vi "启动.vi"   [LabVIEW 2016]
uses:
  <vilib>/addons/WireFlow/_WF_ProgressBar.llb/MessageTextType.ctl
  <vilib>/addons/WireFlow/_WF_ProgressBar.llb/WindowBehavior.ctl
  <vilib>/addons/WireFlow/_WF_ProgressBar.llb/ProgressBar_WireFlow.lvclass
  API/update/update.lvlib
types:
  T1 = typedef "ProgressBar_WireFlow.lvclass/WindowBehavior.ctl" = enum16{"No change", "Modal", "Floating"}
  T2 = typedef "ProgressBar_WireFlow.lvclass/MessageTextType.ctl" = enum16{"Title", "General", "Current item"}
  T3 = enum32{"Invalid", "Standard", "Closed", "Hidden", "Minimized", "Maximized"}
  T4 = cluster{"host":string, "port":u16, "user":string, "password":string, "远端地址":string}
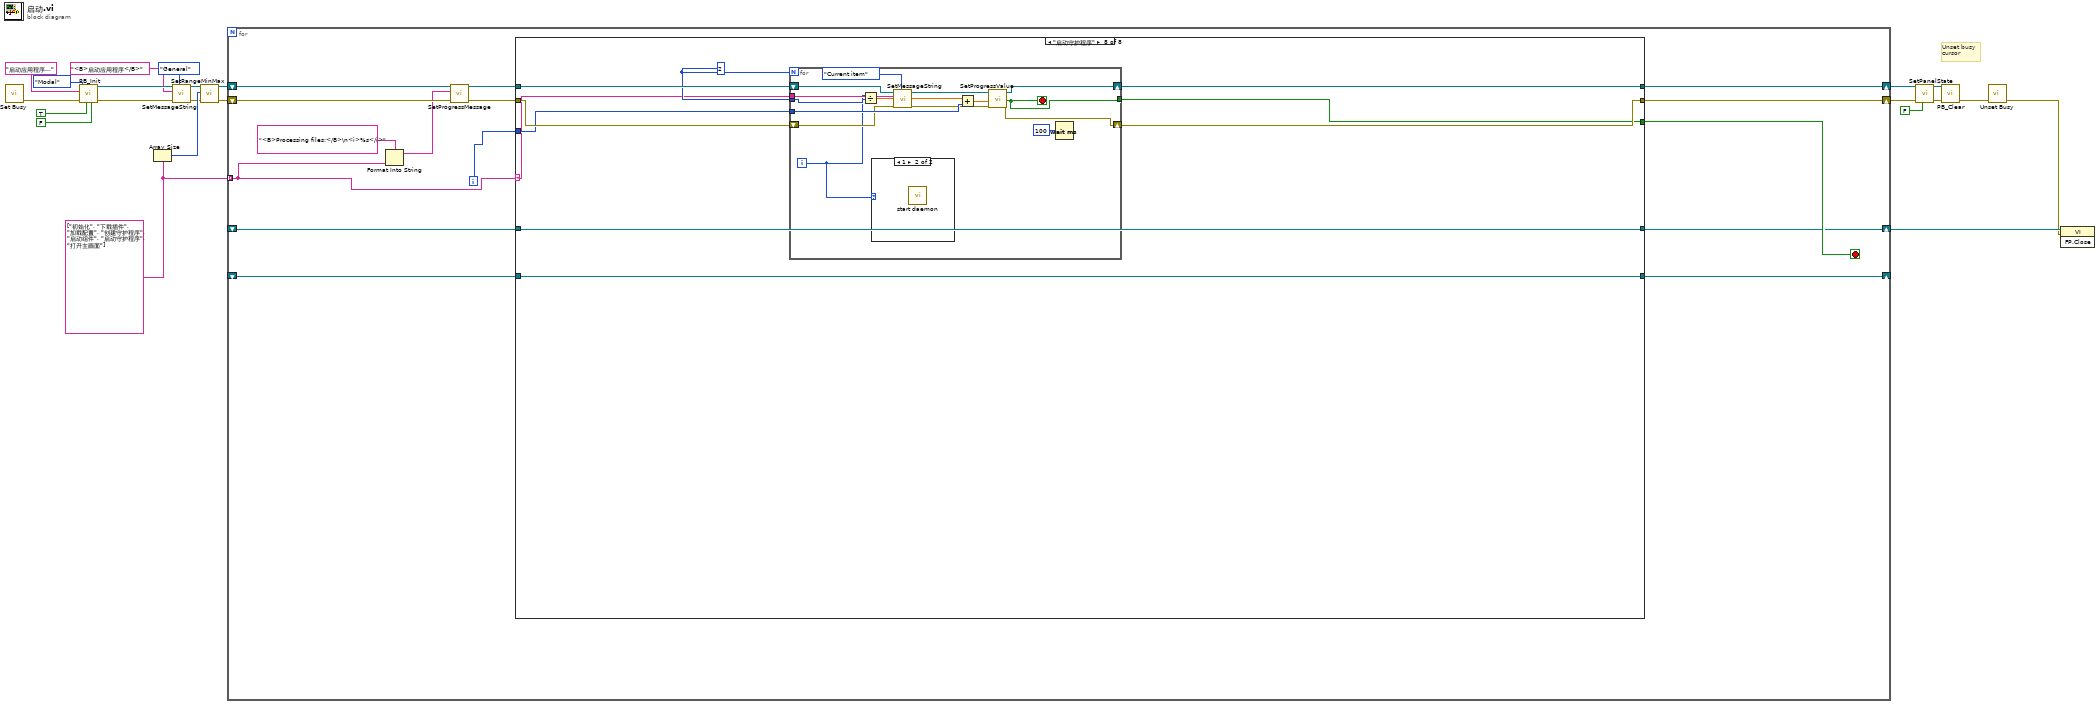
[diagram p0: block diagram]
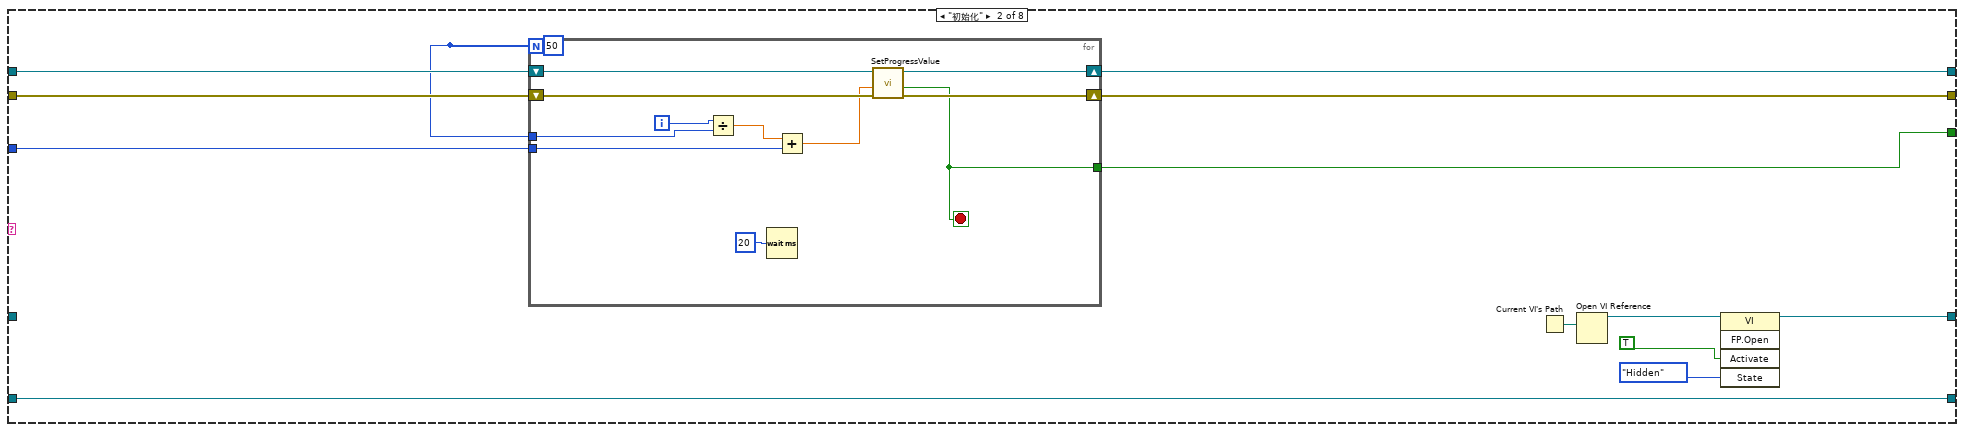
[diagram p3: hidden frame]
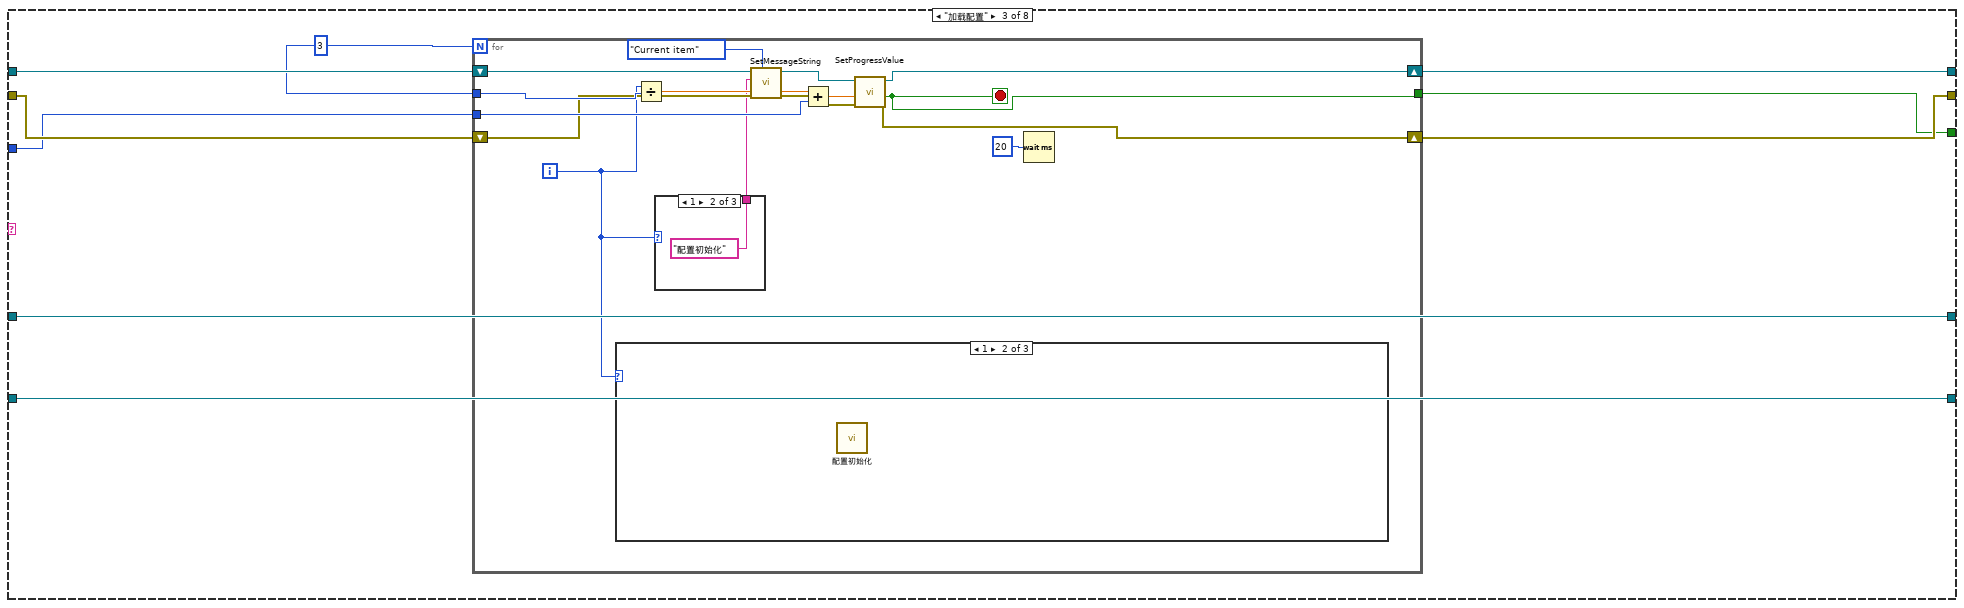
[diagram p4: hidden frame]
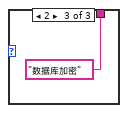
[diagram p6: hidden frame]
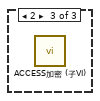
[diagram p8: hidden frame]
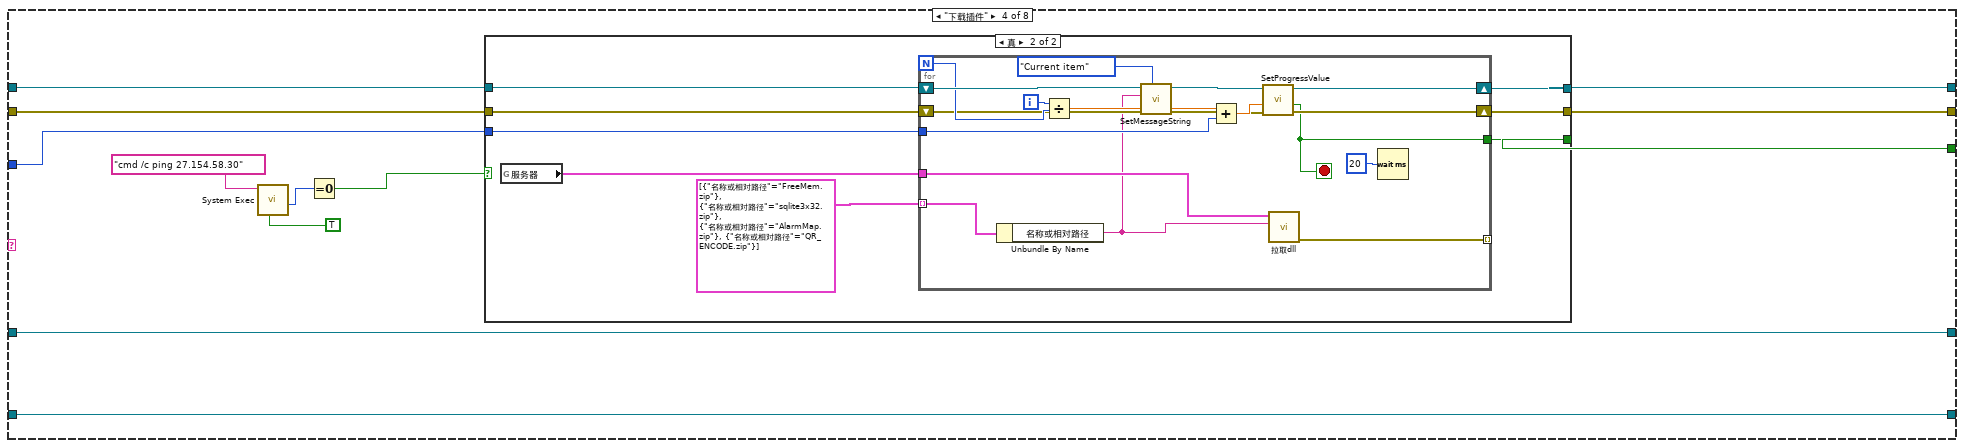
[diagram p9: hidden frame]
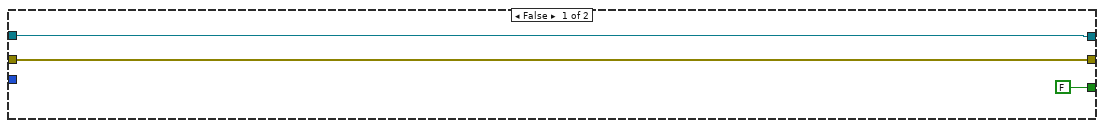
[diagram p10: hidden frame]
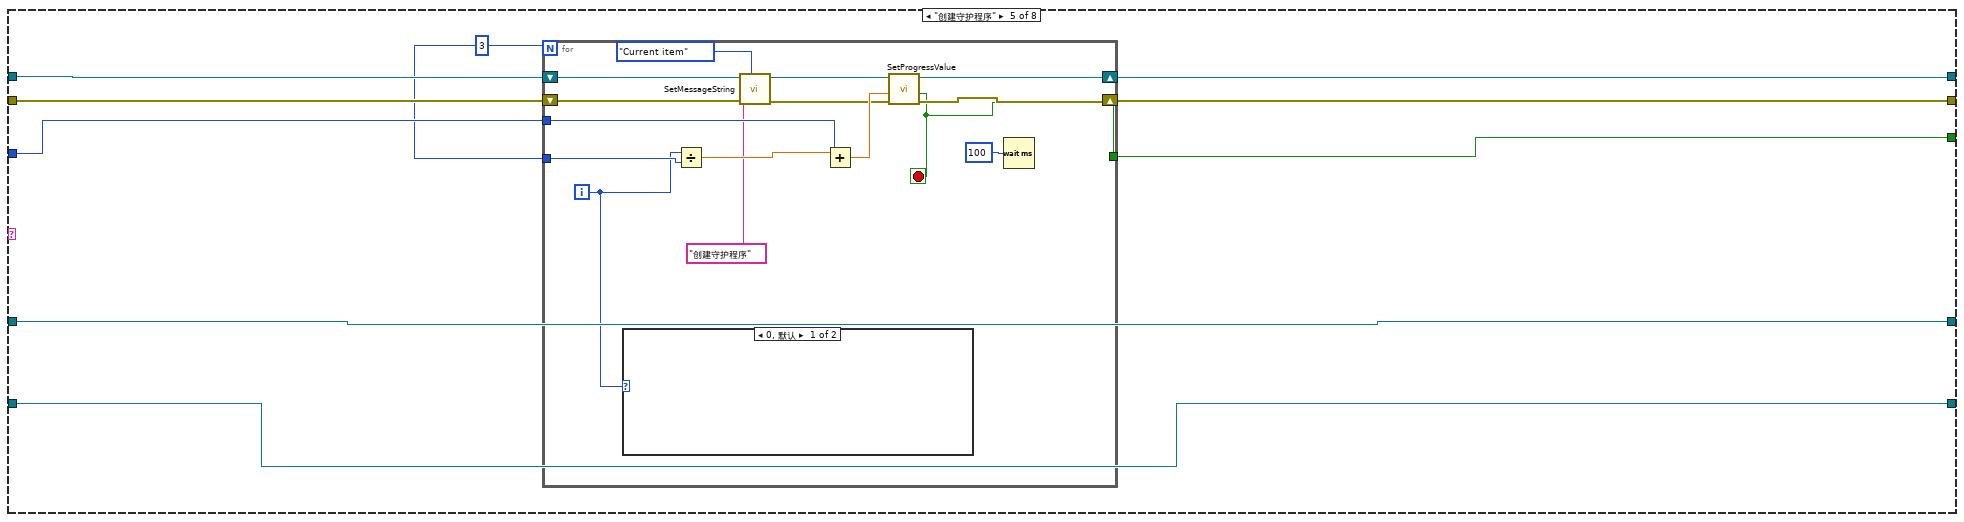
[diagram p11: hidden frame]
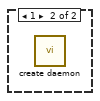
[diagram p12: hidden frame]
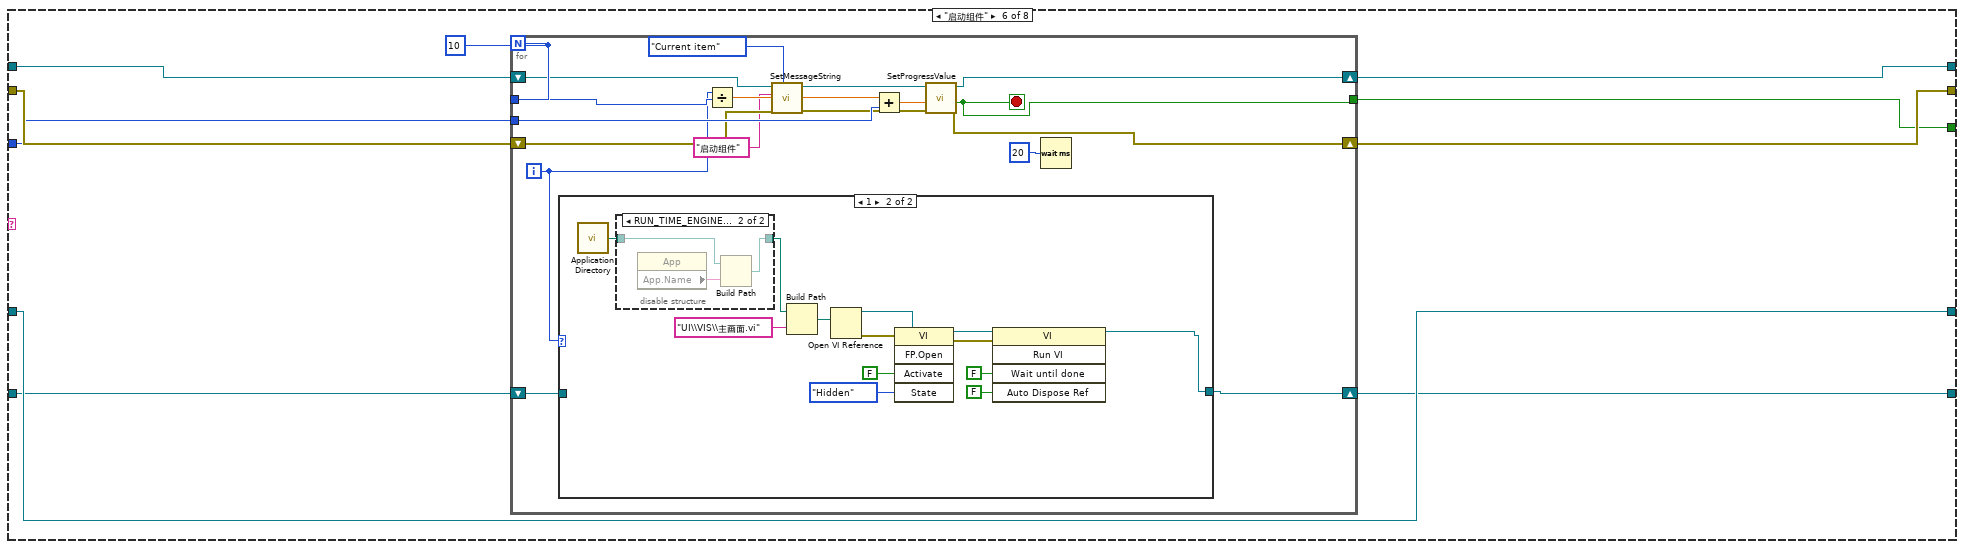
[diagram p13: hidden frame]
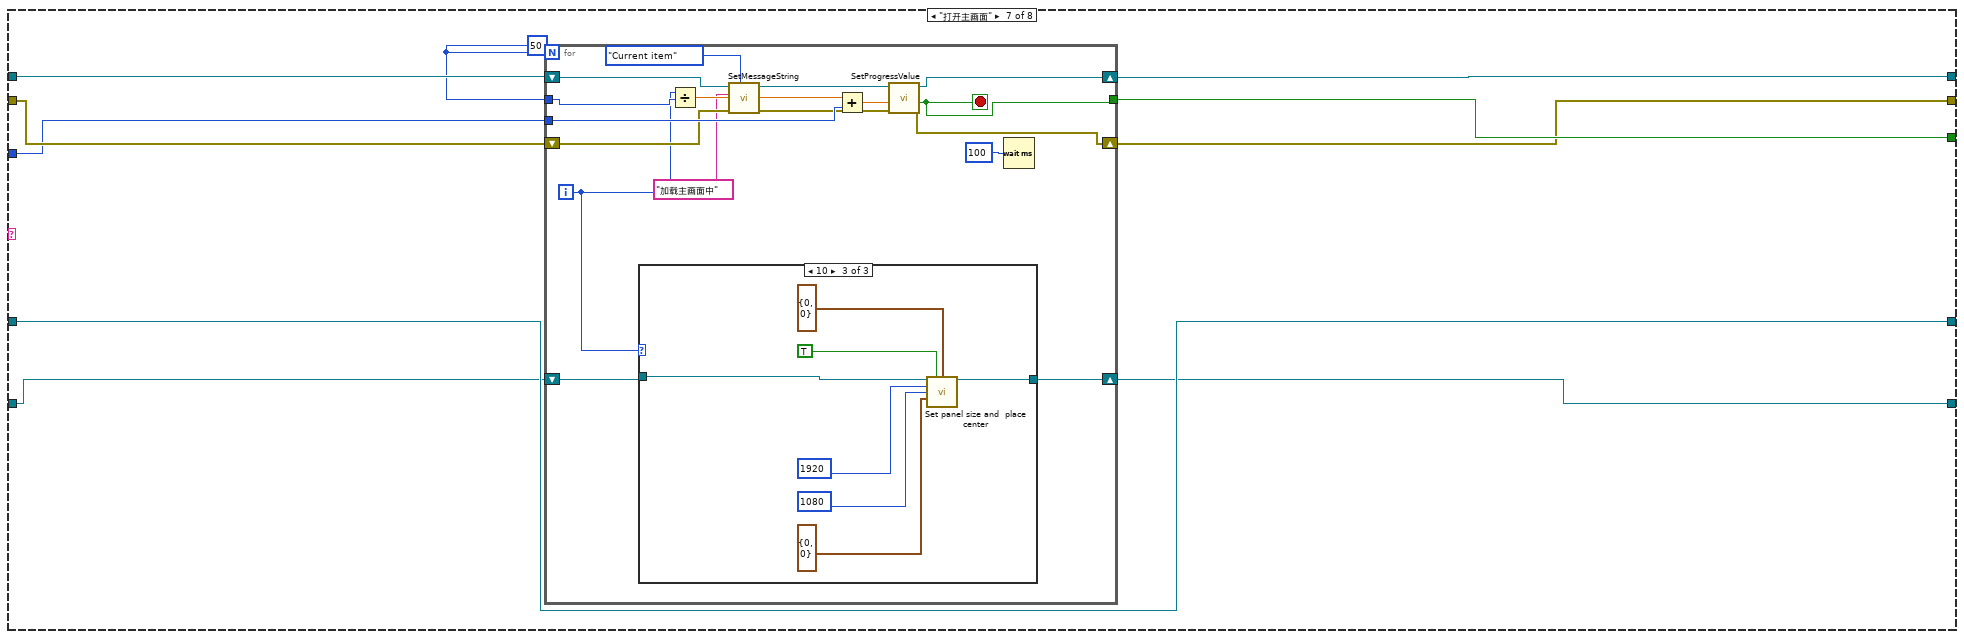
[diagram p16: hidden frame]
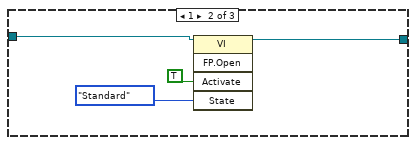
[diagram p18: hidden frame]
diagram:
  w18 = string[] ["初始化", "下载插件", "加载配置", "创建守护程序", "启动组件", "启动守护程序", "打开主画面"]
  # "Unset busy cursor"
  n1 = call <vilib>:"Set Busy.vi"() -> ("error out"=w8:errorcluster)  [unwired: 10 in, 1 out]
  n2 = call <vilib>:"PB_Init.vi"("Cancel button active? (False)"=FALSE ("Cancel active?"), "Open (TRUE)"=TRUE, "error in (no error)"=w8, "Window behavior (No change)"=WindowBehavior."Modal", "title (\"Progress\")"="启动应用程序..." ("title (\"Progress\")")) -> ("error out"=w12:errorcluster, "WF-ProgressBar out"=w14:refnum<class "ProgressBar_WireFlow.lvclass">)  [unwired: 5 in]
  n3 = Array Size(array=w18) -> (size(s)=w19:i32)
  n4 = call-dynamic "SetMessageString.vi"("message field"=MessageTextType."General", "error in (no error)"=w12, "Message"="<B>启动应用程序</B>", "WF-ProgressBar in"=w14) -> ("error out"=w11:errorcluster, "WF-ProgressBar out"=w13:refnum<class "ProgressBar_WireFlow.lvclass">)  [unwired: 6 in]
  n5 = call-dynamic "SetRangeMinMax.vi"("error in (no error)"=w11, "Max (1)"=w19, "WF-ProgressBar in"=w13) -> ("error out"=w4:errorcluster, "WF-ProgressBar out"=w5:refnum<class "ProgressBar_WireFlow.lvclass">)  [unwired: 7 in]
  n6 = for {
    shift-right: [w36] -> w20
    shift-left: w5 -> [w38]
    shift-right: [w30] -> w21
    shift-left: w4 -> [w35]
    tunnel: w18 -> [w28] mode=indexing
    shift-right: [w27] -> w3
    shift-left: _ -> [w26]
    shift-right: [w25] -> _
    shift-left: _ -> [w24]
    i -> [w31]
    stop <- w29 stop-if-true
    n7 = Format Into String(format string="<B>Processing files:</B>\n<i>%s</i>", w28) -> (resulting string=w32:string)  [unwired: 2 in, 1 out]
    n8 = call-dynamic "SetProgressMessage.vi"("error in (no error)"=w35, "Message"=w32, "WF-ProgressBar in"=w38) -> ("error out"=w34:errorcluster, "WF-ProgressBar out"=w37:refnum<class "ProgressBar_WireFlow.lvclass">)  [unwired: 6 in, 1 out]
    n9 = case shown="\"启动守护程序\"" w28 {
      selector: w28 -> [_ _ _ _ _ _ _ w242]
      tunnel: w37 -> [w42 w55 w75 w104 w142 w167 w212 w251]
      tunnel: [w42 w54 w74 w103 w141 w166 w211 w250] -> w36
      tunnel: w34 -> [w41 w53 w73 w102 w140 w165 w210 w249]
      tunnel: w31 -> [_ w52 w72 w101 w139 w164 w209 w248]
      tunnel: [w41 w50 w70 w100 w137 w162 w205 w246] -> w30
      tunnel: [_ w49 w69 w99 w136 w161 w207 w245] -> w29
      tunnel: [w40 w44 w68 w98 w135 w160 w206 w243] -> w27
      tunnel: w26 -> [w40 _ w68 w98 w135 w160 w206 w243]
      tunnel: [w39 w43 w67 w97 w134 w159 w203 w244] -> w25
      tunnel: w24 -> [w39 w43 w67 w97 w134 w158 w204 w244]
      frame Default {
      }
      frame "初始化" {
        w51 = 50
        n10 = for {
          N: w51 -> [_]
          tunnel: w52 -> [w61]
          shift-right: [w65] -> w54
          shift-left: w55 -> [w66]
          shift-right: [w57] -> w50
          shift-left: w53 -> [w64]
          tunnel: w51 -> [w58]
          tunnel: [w56] -> w49
          i -> [w63]
          stop <- w56 stop-if-true
          n11 = Divide(x=w63, y=w58) -> (x/y=w62:dbl)
          n12 = Wait (ms)(milliseconds to wait=u32 20) -> ()  [unwired: 1 out]
          n13 = Add(x=w62, y=w61) -> (x+y=w60:dbl)
          n14 = call-dynamic "SetProgressValue.vi"("error in (no error)"=w64, "Value"=w60, "WF-ProgressBar in"=w66) -> ("error out"=w57:errorcluster, "cancelled?"=w56:bool, "WF-ProgressBar out"=w65:refnum<class "ProgressBar_WireFlow.lvclass">)  [unwired: 6 in]
        }
        n15 = Current VI's Path() -> (path=w46:path)
        n16 = Open VI Reference(vi path=w46) -> (vi reference=w45:refnum<vi>)  [unwired: 5 in, 1 out]
        n17 = invoke class="VI" method="FP.Open"(reference=w45, "Activate"=TRUE ("激活？"), "State"=T3."Hidden" ("状态")) -> (reference out=w44:refnum<vi>)  [unwired: 2 in, 4 out]
      }
      frame "加载配置" {
        w71 = 3
        n18 = for {
          N: w71 -> [_]
          tunnel: w72 -> [w87]
          shift-right: [w89] -> w74
          shift-left: w75 -> [w90]
          shift-right: [w83] -> w70
          shift-left: w73 -> [w80]
          tunnel: w71 -> [w84]
          tunnel: [w82] -> w69
          i -> [w77]
          stop <- w82 stop-if-true
          n19 = case shown="1" w77 {
            frame 0, Default {
            }
            frame 1 {
              n20 = call "配置初始化.vi"() -> ()  [unwired: 11 in, 1 out]
            }
            frame 2 {
              n21 = call "ACCESS加密 (子VI).vi"() -> ()  [unwired: 11 in, 1 out]
            }
          }
          n22 = Divide(x=w77, y=w84) -> (x/y=w88:dbl)
          n23 = case shown="1" w77 {
            tunnel: [_ "配置初始化" "数据库加密"] -> w76
            frame 0, Default {
            }
            frame 1 {
            }
            frame 2 {
            }
          }
          n24 = call-dynamic "SetMessageString.vi"("message field"=MessageTextType."Current item", "error in (no error)"=w80, "Message"=w76, "WF-ProgressBar in"=w90) -> ("error out"=w79:errorcluster, "WF-ProgressBar out"=w81:refnum<class "ProgressBar_WireFlow.lvclass">)  [unwired: 6 in]
          n25 = Add(x=w88, y=w87) -> (x+y=w86:dbl)
          n26 = call-dynamic "SetProgressValue.vi"("error in (no error)"=w79, "Value"=w86, "WF-ProgressBar in"=w81) -> ("error out"=w83:errorcluster, "cancelled?"=w82:bool, "WF-ProgressBar out"=w89:refnum<class "ProgressBar_WireFlow.lvclass">)  [unwired: 6 in]
          n27 = Wait (ms)(milliseconds to wait=u32 20) -> ()  [unwired: 1 out]
        }
      }
      frame "下载插件" {
        n28 = call <vilib>:"System Exec.vi"("run minimized? (F)"=TRUE, "command line"="cmd /c ping 27.154.58.30") -> ("return code"=w94:i32)  [unwired: 6 in, 3 out]
        n29 = Equal To 0?(x=w94) -> (x = 0?=w93:bool)
        n30 = case shown="真" w93 {
          tunnel: w104 -> [w107 w115]
          tunnel: [w107 w114] -> w103
          tunnel: w102 -> [w106 w113]
          tunnel: w101 -> [_ w112]
          tunnel: [w106 w111] -> w100
          tunnel: [FALSE ("cancelled?") w110] -> w99
          frame False {
          }
          frame True {
            n31 = global read "系统设置全局变量.vi" "服务器"() -> (w108:T4)
            n32 = for {
              N -> [w122]
              tunnel: w112 -> [w129]
              shift-right: [w132] -> w114
              shift-left: w115 -> [w133]
              shift-right: [w126] -> w111
              shift-left: w113 -> [w119]
              tunnel: [w125] -> w110
              tunnel: cluster{"名称或相对路径":string}[] [{"名称或相对路径"="FreeMem.zip"}, {"名称或相对路径"="sqlite3x32.zip"}, {"名称或相对路径"="AlarmMap.zip"}, {"名称或相对路径"="QR_ENCODE.zip"}] -> [w124] mode=indexing
              tunnel: w108 -> [w123]
              tunnel: [w121] -> _ mode=indexing
              i -> [w131]
              stop <- w125 stop-if-true
              n33 = Unbundle By Name(w124) -> ("名称或相对路径"=w116:string)
              n34 = Divide(x=w131, y=w122) -> (x/y=w130:dbl)
              n35 = call-dynamic "SetMessageString.vi"("message field"=MessageTextType."Current item", "error in (no error)"=w119, "Message"=w116, "WF-ProgressBar in"=w133) -> ("error out"=w118:errorcluster, "WF-ProgressBar out"=w120:refnum<class "ProgressBar_WireFlow.lvclass">)  [unwired: 6 in]
              n36 = Add(x=w130, y=w129) -> (x+y=w128:dbl)
              n37 = call-dynamic "SetProgressValue.vi"("error in (no error)"=w118, "Value"=w128, "WF-ProgressBar in"=w120) -> ("error out"=w126:errorcluster, "cancelled?"=w125:bool, "WF-ProgressBar out"=w132:refnum<class "ProgressBar_WireFlow.lvclass">)  [unwired: 6 in]
              n38 = call "拉取dll.vi"("名称或相对路径"=w116, "服务器"=w123) -> ("error out"=w121:errorcluster)  [unwired: 9 in]
              n39 = Wait (ms)(milliseconds to wait=u32 20) -> ()  [unwired: 1 out]
            }
          }
        }
      }
      frame "创建守护程序" {
        w138 = 3
        n40 = for {
          N: w138 -> [_]
          tunnel: w139 -> [w154]
          shift-right: [w156] -> w141
          shift-left: w142 -> [w157]
          shift-right: [w150] -> w137
          shift-left: w140 -> [w147]
          tunnel: w138 -> [w151]
          tunnel: [w149] -> w136
          i -> [w145]
          stop <- w149 stop-if-true
          n41 = case shown="0, 默认" w145 {
            frame 0, Default {
            }
            frame 1 {
              n42 = call "create daemon.vi"() -> ()  [unwired: 11 in, 1 out]
            }
          }
          n43 = Divide(x=w145, y=w151) -> (x/y=w155:dbl)
          n44 = call-dynamic "SetMessageString.vi"("message field"=MessageTextType."Current item", "error in (no error)"=w147, "Message"="创建守护程序", "WF-ProgressBar in"=w157) -> ("error out"=w146:errorcluster, "WF-ProgressBar out"=w148:refnum<class "ProgressBar_WireFlow.lvclass">)  [unwired: 6 in]
          n45 = Add(x=w155, y=w154) -> (x+y=w153:dbl)
          n46 = call-dynamic "SetProgressValue.vi"("error in (no error)"=w146, "Value"=w153, "WF-ProgressBar in"=w148) -> ("error out"=w150:errorcluster, "cancelled?"=w149:bool, "WF-ProgressBar out"=w156:refnum<class "ProgressBar_WireFlow.lvclass">)  [unwired: 6 in]
          n47 = Wait (ms)(milliseconds to wait=u32 100) -> ()  [unwired: 1 out]
        }
      }
      frame "启动组件" {
        w163 = 10
        n48 = for {
          N: w163 -> [_]
          tunnel: w164 -> [w181]
          shift-right: [w183] -> w166
          shift-left: w167 -> [w184]
          shift-right: [w177] -> w162
          shift-left: w165 -> [w171]
          tunnel: w163 -> [w178]
          tunnel: [w176] -> w161
          shift-right: [w175] -> w159
          shift-left: w158 -> [w173]
          i -> [w174]
          stop <- w176 stop-if-true
          n49 = case shown="1" w174 {
            tunnel: [w185 w193] -> w175
            tunnel: w173 -> [w185 _]
            frame Default {
            }
            frame 1 {
              n50 = call <vilib>:"Application Directory.vi"() -> ("Application Directory"=w195:path)
              n51 = disable-structure shown="RUN_TIME_ENGINE==True" {
                disable-tunnel: w195 -> [w199 w202]
                disable-tunnel: [w199 w200] -> w194
                frame condition #0 (active) {
                }
                frame condition #1 {
                  n52 = property class="App"() -> ("App.Name"=w201:string)  [unwired: 2 in, 2 out]
                  n53 = Build Path(base path=w202, name or relative path=w201) -> (appended path=w200:path)
                }
              }
              n54 = Build Path(base path=w194, name or relative path="UI\\VIS\\主画面.vi" ("名称或相对路径")) -> (appended path=w186:path)
              n55 = Open VI Reference(vi path=w186) -> (vi reference=w192:refnum<vi>, error out=w190:errorcluster)  [unwired: 5 in]
              n56 = invoke class="VI" method="FP.Open"(reference=w192, error in=w190, "Activate"=FALSE ("激活？"), "State"=T3."Hidden" ("状态")) -> (reference out=w191:refnum<vi>, error out=w189:errorcluster)  [unwired: 1 in, 3 out]
              n57 = invoke class="VI" method="Run VI"(reference=w191, error in=w189, "Wait until done"=FALSE ("结束前等待"), "Auto Dispose Ref"=FALSE ("自动销毁引用")) -> (reference out=w193:refnum<vi>)  [unwired: 1 in, 4 out]
            }
          }
          n58 = Divide(x=w174, y=w178) -> (x/y=w182:dbl)
          n59 = call-dynamic "SetMessageString.vi"("message field"=MessageTextType."Current item", "error in (no error)"=w171, "Message"="启动组件", "WF-ProgressBar in"=w184) -> ("error out"=w170:errorcluster, "WF-ProgressBar out"=w172:refnum<class "ProgressBar_WireFlow.lvclass">)  [unwired: 6 in]
          n60 = Add(x=w182, y=w181) -> (x+y=w180:dbl)
          n61 = call-dynamic "SetProgressValue.vi"("error in (no error)"=w170, "Value"=w180, "WF-ProgressBar in"=w172) -> ("error out"=w177:errorcluster, "cancelled?"=w176:bool, "WF-ProgressBar out"=w183:refnum<class "ProgressBar_WireFlow.lvclass">)  [unwired: 6 in]
          n62 = Wait (ms)(milliseconds to wait=u32 20) -> ()  [unwired: 1 out]
        }
      }
      frame "打开主画面" {
        w208 = 50
        n63 = for {
          N: w208 -> [_]
          tunnel: w209 -> [w226]
          shift-right: [w228] -> w211
          shift-left: w212 -> [w229]
          shift-right: [w222] -> w205
          shift-left: w210 -> [w218]
          tunnel: w208 -> [w223]
          tunnel: [w221] -> w207
          shift-right: [w213] -> w203
          shift-left: w204 -> [w214]
          i -> [w215]
          stop <- w221 stop-if-true
          n64 = case shown="10" w215 {
            tunnel: w214 -> [w230 w232 w235]
            tunnel: [w230 w231 w236] -> w213
            frame 0, Default {
            }
            frame 1 {
              n65 = invoke class="VI" method="FP.Open"(reference=w232, "Activate"=TRUE ("激活？"), "State"=T3."Standard" ("状态")) -> (reference out=w231:refnum<vi>)  [unwired: 2 in, 4 out]
            }
            frame 10 {
              n66 = call "Set panel size and  place center.vi"("VI引用句柄"=w235, "Close Reference (false)"=TRUE, "FP.WinOrigin in(H & V)"=cluster{"Horizontal":i16, "Vertical":i16} {"Horizontal"=0, "Vertical"=0}, "Panel Width"=1920, "Panel Height"=1080, "FP.Origin in(H & V)"=cluster{"Horizontal":i16, "Vertical":i16} {"Horizontal"=0, "Vertical"=0}) -> ("Application or VI Refnum"=w236:refnum<vi>)  [unwired: 8 in, 1 out]
            }
          }
          n67 = Divide(x=w215, y=w223) -> (x/y=w227:dbl)
          n68 = call-dynamic "SetMessageString.vi"("message field"=MessageTextType."Current item", "error in (no error)"=w218, "Message"="加载主画面中", "WF-ProgressBar in"=w229) -> ("error out"=w217:errorcluster, "WF-ProgressBar out"=w220:refnum<class "ProgressBar_WireFlow.lvclass">)  [unwired: 6 in]
          n69 = Add(x=w227, y=w226) -> (x+y=w225:dbl)
          n70 = call-dynamic "SetProgressValue.vi"("error in (no error)"=w217, "Value"=w225, "WF-ProgressBar in"=w220) -> ("error out"=w222:errorcluster, "cancelled?"=w221:bool, "WF-ProgressBar out"=w228:refnum<class "ProgressBar_WireFlow.lvclass">)  [unwired: 6 in]
          n71 = Wait (ms)(milliseconds to wait=u32 100) -> ()  [unwired: 1 out]
        }
      }
      frame "启动守护程序" {
        w247 = 2
        n72 = for {
          N: w247 -> [_]
          tunnel: w248 -> [w263]
          shift-right: [w265] -> w250
          shift-left: w251 -> [w266]
          shift-right: [w259] -> w246
          shift-left: w249 -> [w256]
          tunnel: w247 -> [w260]
          tunnel: [w258] -> w245
          tunnel: w242 -> [w254]
          i -> [w252]
          stop <- w258 stop-if-true
          n73 = Divide(x=w252, y=w260) -> (x/y=w264:dbl)
          n74 = case shown="1" w252 {
            frame 0, Default {
            }
            frame 1 {
              n75 = call "start daemon.vi"() -> ()  [unwired: 11 in, 1 out]
            }
          }
          n76 = call-dynamic "SetMessageString.vi"("message field"=MessageTextType."Current item", "error in (no error)"=w256, "Message"=w254, "WF-ProgressBar in"=w266) -> ("error out"=w255:errorcluster, "WF-ProgressBar out"=w257:refnum<class "ProgressBar_WireFlow.lvclass">)  [unwired: 6 in]
          n77 = Add(x=w264, y=w263) -> (x+y=w262:dbl)
          n78 = call-dynamic "SetProgressValue.vi"("error in (no error)"=w255, "Value"=w262, "WF-ProgressBar in"=w257) -> ("error out"=w259:errorcluster, "cancelled?"=w258:bool, "WF-ProgressBar out"=w265:refnum<class "ProgressBar_WireFlow.lvclass">)  [unwired: 6 in]
          n79 = Wait (ms)(milliseconds to wait=u32 100) -> ()  [unwired: 1 out]
        }
      }
    }
  }
  n80 = call-dynamic "SetPanelState.vi"("State (T = Open)"=FALSE, "error in (no error)"=w21, "WF-ProgressBar in"=w20) -> ("error out"=w15:errorcluster, "WF-ProgressBar out"=w16:refnum<class "ProgressBar_WireFlow.lvclass">)  [unwired: 7 in]
  n81 = call-dynamic "PB_Clear.vi"("error in (no error)"=w15, "WF-ProgressBar in"=w16) -> ("error out"=w7:errorcluster)  [unwired: 8 in, 1 out]
  n82 = call <vilib>:"Unset Busy.vi"("error in (no error)"=w7) -> ("error out"=w2:errorcluster)  [unwired: 10 in]
  n83 = invoke class="VI" method="FP.Close"(reference=w3, error in=w2) -> ()  [unwired: 1 in, 3 out]
